vi "Log_creation.vi"(4 "VM's path":path, 6 "Target File Path":path, 7 "Log file path":path, 8 "error in":errorcluster, 9 "Item Names":string[](array[string]), 10 "Listbox Target":i32[](listbox), 11 "VM name":string) -> (0 "error out":errorcluster)   [LabVIEW 2015]
panel:
  out "current time":timestamp
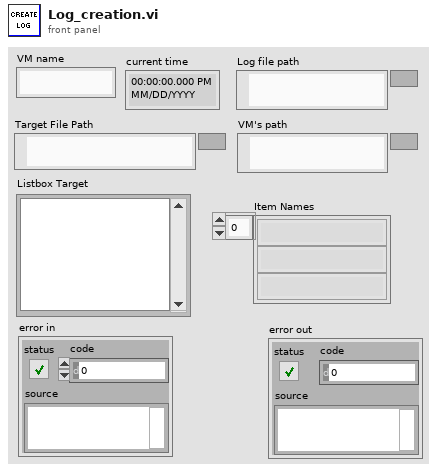
[diagram p1: front panel]
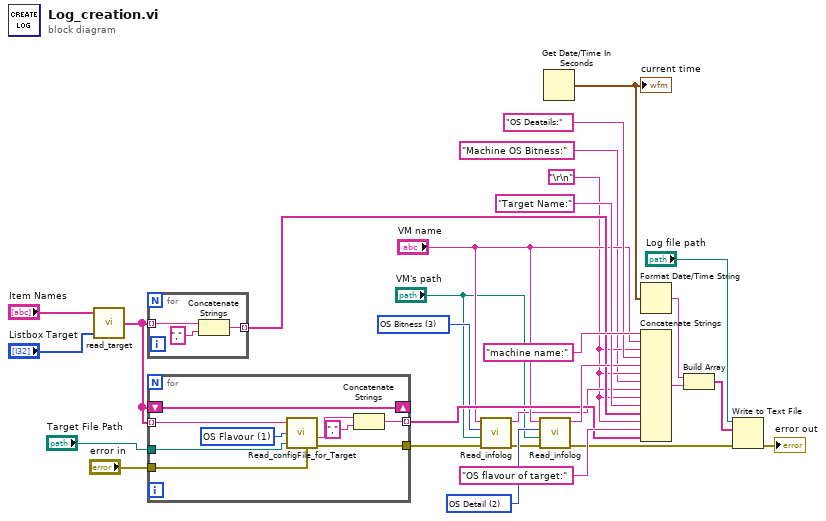
[diagram p0: block diagram]
diagram:
  w13 = u16 3 items=["VM Name", "VMX Path", "OS Detail", "OS Bitness"] ("Ring")
  w10 = "\r\n"
  w28 = u16 2 items=["VM Name", "VMX Path", "OS Detail", "OS Bitness"] ("Ring")
  n1 = call "read_target.vi"("Listbox  Target"="Listbox Target", "Item Names"="Item Names") -> ("Array"=w16:string[])
  n2 = for {
    tunnel: w16 -> [w31] mode=indexing
    tunnel: [w30] -> w15 mode=indexing
    n3 = Concatenate Strings(w31, "," ("string")) -> (w30:string)
  }
  n4 = for {
    tunnel: w16 -> [w38] mode=indexing
    shift-right: [w40] -> _
    shift-left: w16 -> [w40]
    tunnel: [w35] -> w14 mode=indexing
    tunnel: [w34] -> w6
    tunnel: "error in" -> [w33]
    tunnel: "Target File Path" -> [w32]
    w39 = u16 1 items=["Target Nmae", "OS Flavour", "Filter  Rates", "Avoid Rates"] ("Ring 2")
    n5 = call "Read_configFile_for_Target.vi"("error in"=w33, "Target File Path"=w32, "Ring 2"=w39, "Target Name"=w38) -> ("error out"=w34:errorcluster, "selected target"=w37:string)  [unwired: 3 in]
    n6 = Concatenate Strings(w37, "," ("string")) -> (w35:string)
  }
  n7 = call "Read_infolog.vi"("vm name"="VM name", "Details of vm"=w13, "VM's path"="VM's path", "error in"=w6) -> ("VMX Path details"=w11:string, "error out"=w8:errorcluster)  [unwired: 5 in]
  n8 = call "Read_infolog.vi"("vm name"="VM name", "Details of vm"=w28, "VM's path"="VM's path", "error in"=w8) -> ("VMX Path details"=w19:string, "error out"=w7:errorcluster)  [unwired: 5 in]
  n9 = Get Date/Time In Seconds() -> (seconds since 1Jan1904=w26:timestamp)
  "current time" <- w26
  n10 = Format Date/Time String(seconds (now)=w26) -> (date/time string=w25:string)  [unwired: 2 in]
  n11 = Concatenate Strings("machine name:", "VM name", w10, "OS Deatails:", w19, w10, "Machine OS Bitness:", w11, w10, "Target Name:", w15, w10, "OS flavour of target:", w14) -> (w23:string)
  n12 = Build Array(w25, w23) -> (w27:string[])
  n13 = Write to Text File(file (use dialog)="Log file path", text=w27, error in=w7) -> (error out=→"error out":errorcluster)  [unwired: 1 in, 2 out]
